vi "ExCircularNframeTime.vi"() -> ()   [LabVIEW 2010]
panel:
  in  "Timing Mode":u32(ring)=1 items=["N/A", "Timed Mode/Free run", "Trigger First (only PM)", "Strobed/Ext Sync", "Bulb Mode (PM only)", "Variable Timed mode (PM only)", "Flash Mode (only some PM)"]
  in  "Number of Images":u32=1 min=1 step=1
  in  "Intensifier":bool
  in  "Temperature":dbl=-10.0 format="%.2f"
  in  "Exposure":dbl min=0.0 step=0.001 format="%.3f"
  out "error out":errorcluster
  in  "error in (no error)":errorcluster
  # "ExCircularNframeTime:\nThis example collects, displays, and saves in \na .r3b file the number of images selected. This \nexample requires the camera have circular \nbuffers capability."
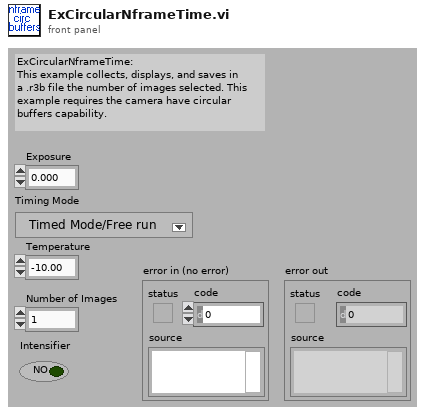
[diagram p1: front panel]
types:
  T1 = cluster{"acquire focus mode":u32, "Exposure":dbl, "Number of Images":u32, "Software accumulation":u32}
  T2 = cluster{"Camera Handle":u32, "Pulser Handle":u32, "File Handle":u32, "Display Handle":u32, "Image Handle":u32}
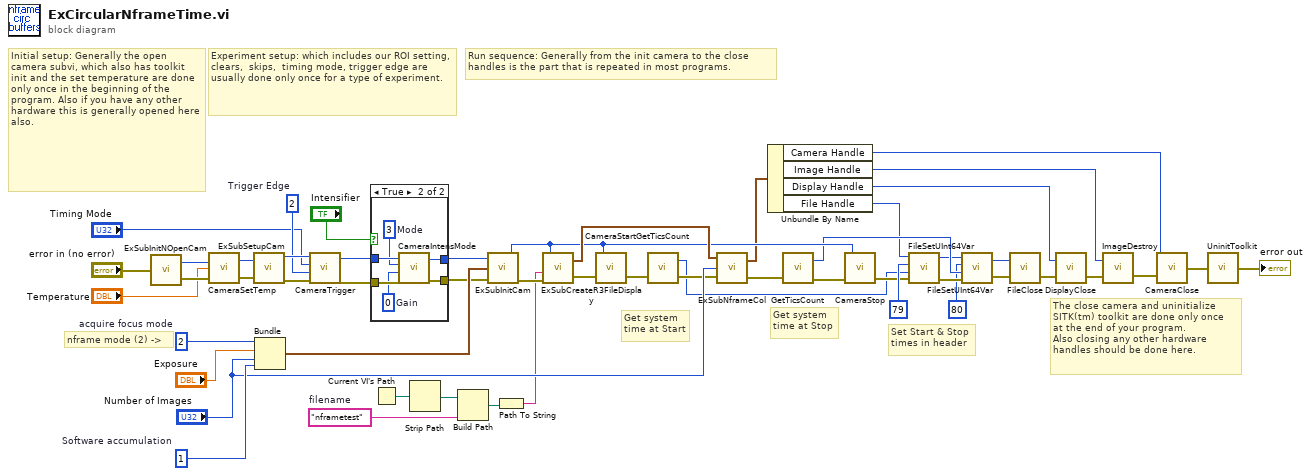
[diagram p0: block diagram]
diagram:
  w43 = u32 2  # Trigger Edge
  w45 = u32 2  # acquire focus mode
  w44 = u32 1  # Software accumulation
  w16 = "nframetest"  # filename
  # "Set Start & Stop\ntimes in header"
  # "Get system\ntime at Stop"
  # "Get system\ntime at Start"
  # "The close camera and uninitialize\nSITK(tm) toolkit are done only once\nat the end of your program.\nAlso closing any other hardware \nhandles should be done here."
  # "Run sequence: Generally from the init camera to the close \nhandles is the part that is repeated in most programs."
  # "Experiment setup: which includes our ROI setting, clears,  skips,  timing mode, trigger edge are usually done only once for a type of experiment."
  # "Initial setup: Generally the open camera subvi, which also has toolkit init and the set temperature are done only once in the beginning of the program. Also if you have any other hardware this is generally opened here also."
  # "nframe mode (2) ->"
  n1 = call "ExSubInitNOpenCam.vi"("error in (no error)"="error in (no error)") -> ("Camera Handle"=w35:u32, "error out"=w34:errorcluster)
  n2 = call <userlib>:"CameraSetTemp.vi"("error in (no error)"=w34, "Temperature"="Temperature", "Camera Handle"=w35) -> ("error out"=w4:errorcluster, "Camera Handle"=w5:u32)
  n3 = call "ExSubSetupCam.vi"("error in (no error)"=w4, "Camera Handle"=w5) -> ("error out"=w47:errorcluster, "Camera Handle"=w48:u32)
  n4 = Bundle("acquire focus mode"=w45, "Exposure"="Exposure", "Number of Images"="Number of Images", "Software accumulation"=w44) -> (w50:T1)  [unwired: 1 in]
  n5 = call <userlib>:"CameraTrigger.vi"("error in"=w47, "Trigger Edge"=w43, "Timing Mode"="Timing Mode", "Camera Handle"=w48) -> ("error out"=w40:errorcluster, "Camera Handle"=w42:u32)
  n6 = case shown="True" "Intensifier" {
    tunnel: w42 -> [w54 w60]
    tunnel: [w54 w59] -> w41
    tunnel: w40 -> [w53 w58]
    tunnel: [w53 w57] -> w39
    frame False {
    }
    frame True {
      w55 = u32 0  # Gain
      w56 = u32 3  # Mode
      n7 = call <userlib>:"CameraIntensMode.vi"("error in"=w58, "Intensifier Gain"=w55, "Mode"=w56, "Camera Handle"=w60) -> ("error out"=w57:errorcluster, "Camera Handle"=w59:u32)
    }
  }
  n8 = Current VI's Path() -> (path=w3:path)
  n9 = Strip Path(path=w3) -> (stripped path=w2:path)  [unwired: 1 out]
  n10 = Build Path(base path=w2, name or relative path=w16) -> (appended path=w17:path)
  n11 = call "ExSubInitCam.vi"("error in (no error)"=w39, "Camera Information"=w50, "Camera Handle"=w41) -> ("error out"=w49:errorcluster, "Camera Handle"=w32:u32)
  n12 = Path To String(path=w17) -> (string=w15:string)
  n13 = call "ExSubCreateR3FileDisplay.vi"("error in (no error)"=w49, "File and Display Name"=w15, "Camera Handle"=w32) -> ("error out"=w46:errorcluster, "Handles Out"=w37:T2)  [unwired: 1 in]
  n14 = call <userlib>:"CameraStart.vi"("error in"=w46, "Camera Handle"=w32) -> ("error out"=w23:errorcluster)  [unwired: 1 out]
  n15 = call <userlib>:"GetTicsCount.vi"("error in"=w23) -> ("Tic Count"=w18:u64, "error out"=w22:errorcluster)
  n16 = call "ExSubNframeCol.vi"("error in (no error)"=w22, "Number of Images"="Number of Images", "Handle Cluster"=w37) -> ("error out"=w29:errorcluster, "Handle Cluster"=w30:T2)
  n17 = Unbundle By Name(w30) -> ("Camera Handle"=w8:u32, "Image Handle"=w10:u32, "Display Handle"=w11:u32, "File Handle"=w25:u32)
  n18 = call <userlib>:"GetTicsCount.vi"("error in"=w29) -> ("Tic Count"=w26:u64, "error out"=w28:errorcluster)
  n19 = call <userlib>:"CameraStop.vi"("error in"=w28, "Camera Handle"=w32) -> ("error out"=w19:errorcluster)  [unwired: 1 out]
  n20 = call <userlib>:"FileSetUInt64Var.vi"("error in"=w19, "Value"=w18, "Parameter ID"=79, "File Handle"=w25) -> ("error out"=w27:errorcluster, "File Handle"=w24:u32)
  n21 = call <userlib>:"FileSetUInt64Var.vi"("error in"=w27, "Value"=w26, "Parameter ID"=80, "File Handle"=w24) -> ("error out"=w1:errorcluster, "File Handle"=w12:u32)
  n22 = call <userlib>:"FileClose.vi"("error in"=w1, "File Handle"=w12) -> ("error out"=w14:errorcluster)
  n23 = call <userlib>:"DisplayClose.vi"("error in"=w14, "Display Handle"=w11) -> ("error out"=w13:errorcluster)
  n24 = call <userlib>:"ImageDestroy.vi"("error in"=w13, "Data handle"=w10) -> ("error out"=w7:errorcluster)
  n25 = call <userlib>:"CameraClose.vi"("error in"=w7, "Camera Handle"=w8) -> ("error out"=w9:errorcluster)
  n26 = call <userlib>:"UninitToolkit.vi"("error in"=w9) -> ("error out"=→"error out":errorcluster)
